vi "读取名称.vi"(8 "error in (no error)":errorcluster caption="错误输入（无错误）", 11 "鸭子库.lvlib:鸭子.lvclass":refnum<class "鸭子.lvclass">) -> (0 "error out":errorcluster caption="错误输出", 2 "名称":string, 3 "鸭子库.lvlib:鸭子.lvclass":refnum<class "鸭子.lvclass">)   [LabVIEW 2022 SP3, in "鸭子库.lvlib" / "鸭子.lvclass"]
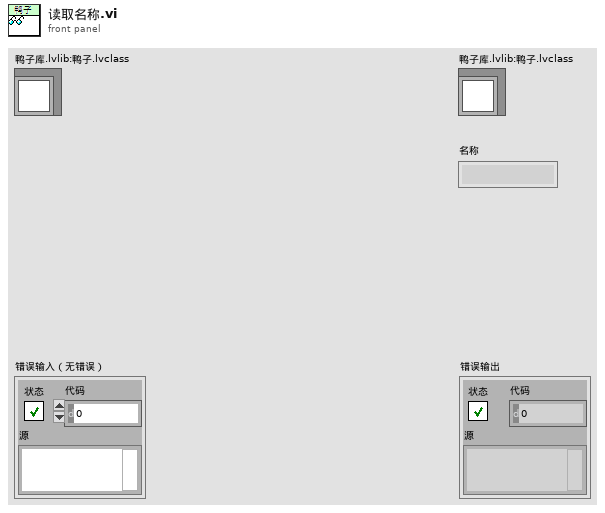
[diagram p1: front panel]
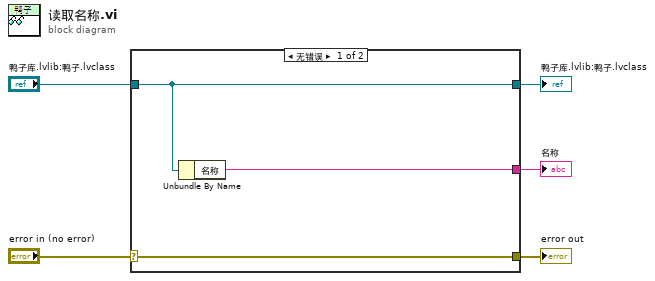
[diagram p0: block diagram]
diagram:
  n1 = case shown="无错误" "error in (no error)" {
    selector: "error in (no error)" -> [w8 w9]
    tunnel: [w8 w9] -> w4
    tunnel: [w7 w10] -> w2
    tunnel: "鸭子库.lvlib:鸭子.lvclass" -> [w7 w10]
    tunnel: [w6 _] -> w1
    frame No Error {
      n2 = Unbundle By Name(w7) -> ("名称"=w6:string)
    }
    frame Error {
    }
  }
  "error out" <- w4
  "鸭子库.lvlib:鸭子.lvclass" <- w2
  "名称" <- w1
